vi "direct_ref_T_sat_p.vi"(8 "Error (Input)":errorcluster, 10 "Saturation pressure in Pa (Input)":dbl, 11 "WorkingPair (Input)":T1={"no_iso"=1, "no_p_sat"=1, "path_db"="D:\\Driesel\\SorpLibLocal\\LabVIEW_wrapper\\data\\json\\sorpproplib_minimalExample.json", "wp_as"="silicagel", "wp_st"="123", "wp_iso"="DubininArctan1", "wp_rf"="water", "rf_rhol"="SaturatedLiquidDensity_EoS1", "no_rhol"=1, "rf_psat"="VaporPressure_EoS1"}) -> (0 "Error (Output)":errorcluster, 3 "Temperature in K (Output)":dbl)   [LabVIEW 2017]
doc: "direct_ref_T_sat_p:\n * -------------------\n *\n * Calculates saturation temperature in K depending on equilibrium pressure p\n * in Pa.\n *\n * Parameters:\n * -----------\n * double p_Pa:\n * Saturation pressure in Pa.\n *\n * const char *path_db:\n * Path to database.\n * const char *wp_as:\n * Name of sorbent.\n * const char *wp_st:\n * Name of sub-type of sorbent.\n * const char *wp_rf:\n * Name of refrigerant.\n * const char *wp_iso:\n * Name of isotherm.\n * int no_iso:\n * ID of isotherm (i.e. when more than one isotherm is available)\n * const char *rf_psat:\n * Name of calculation approach for vapor pressure.\n * int no_p_sat:\n * ID of vapor pressure equation (i.e. when more than one equation is\n * available)\n * const char *rf_rhol:\n * Name of calculation approach for liquid density.\n * int no_rhol:\n * ID of liquid density equation (i.e. when more than one equation is\n * available)\n *\n * Returns:\n * --------\n * double:\n * Equilibrium temperature in K.\n *\n * History:\n * --------\n *12/07/2021, by Jannik Driesel (supervised by Mirko Engelpracht)\n * First implementation."
uses:
  data/win32bit/libsorpPropLib.dll
panel:
  # "Path to database"
  # "Name of sorbent"
  # "Name of sub-type of sorbent"
  # "Name of refrigerant"
  # "Name of isotherm"
  # "ID of isotherm"
  # "Name of calculation approach for vapor pressure"
  # "ID of vapor pressure equation"
  # "Name of calculation approach for liquid density"
  # "ID of liquid density equation"
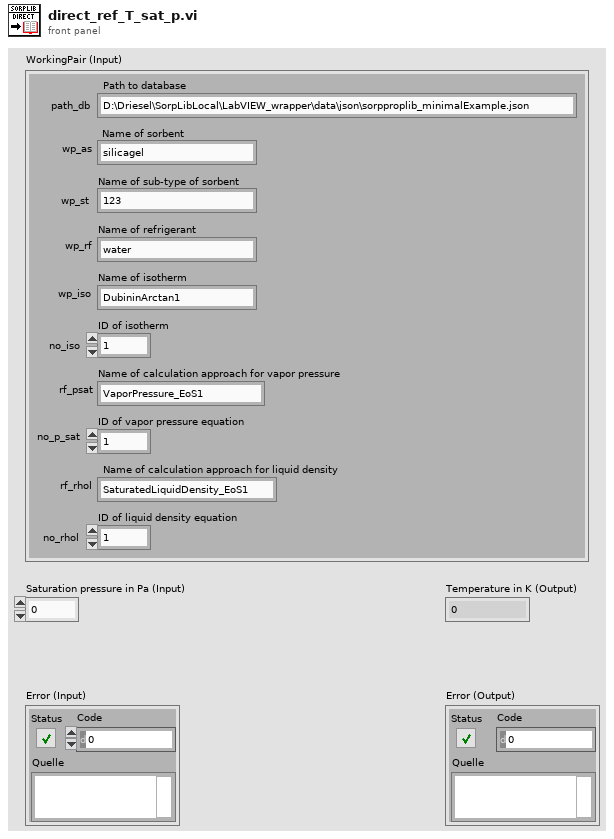
[diagram p1: front panel]
types:
  T1 = cluster{"no_iso":i32, "no_p_sat":i32, "path_db":string, "wp_as":string, "wp_st":string, "wp_iso":string, "wp_rf":string, "rf_rhol":string, "no_rhol":i32, "rf_psat":string}
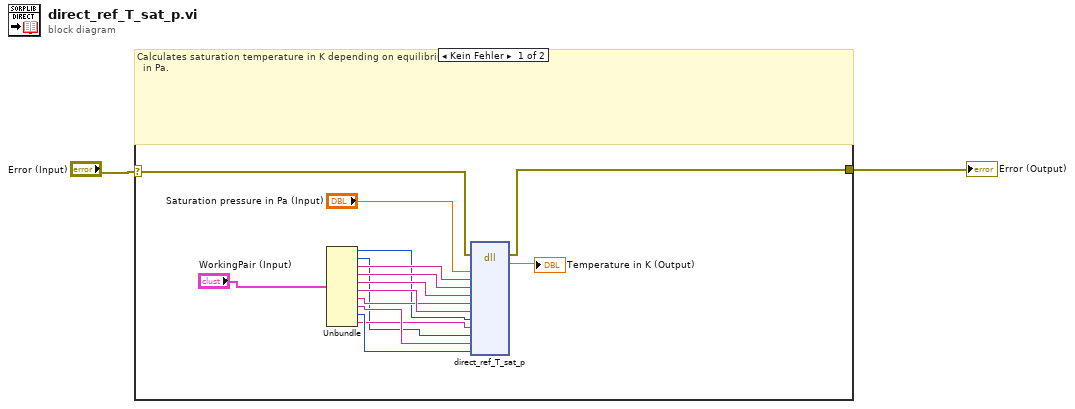
[diagram p0: block diagram]
diagram:
  n1 = case shown="Kein Fehler" "Error (Input)" {
    selector: "Error (Input)" -> [w15 w18]
    tunnel: [w16 w18] -> w2
    frame No Error {
      # "Calculates saturation temperature in K depending on equilibrium pressure p\n  in Pa."
      n2 = Unbundle("WorkingPair (Input)") -> ("no_iso"=w5:i32, "no_p_sat"=w4:i32, "path_db"=w13:string, "wp_as"=w12:string, "wp_st"=w11:string, "wp_iso"=w10:string, "wp_rf"=w9:string, "rf_rhol"=w8:string, "no_rhol"=w7:i32, "rf_psat"=w6:string)
      n3 = dll-call lib="D:/Driesel/SorpLibLocal/LabVIEW_wrapper/data/win32bit/libsorpPropLib.dll" fn="direct_ref_T_sat_p"(error in=w15, "T_K"="Saturation pressure in Pa (Input)", "path_db"=w13, "wp_as"=w12, "wp_st"=w11, "wp_rf"=w9, "wp_iso"=w10, "no_iso"=w5, "rf_psat"=w6, "no_p_sat"=w4, "rf_rhol"=w8, "no_rhol"=w7) -> (error out=w16:errorcluster, "T_sat_K"=→"Temperature in K (Output)":dbl)  [unwired: 13 in, 1 out]
    }
    frame Error {
      # "Error - No calculations"
    }
  }
  "Error (Output)" <- w2
